vi "Unsubscribe.vi"(7 "Close if last?":bool, 8 "error in (no error)":errorcluster, 10 "Receivers Enqueuer":refnum<class "Message Enqueuer.lvclass">, 11 "Pub Sub Message Channel in":refnum<class "Pub Sub Message Channel.lvclass">) -> (0 "error out":errorcluster, 3 "Pub Sub Message Channel out":refnum<class "Pub Sub Message Channel.lvclass">)   [LabVIEW 2020, in "Actor Pub Sub Channels.lvlib" / "Pub Sub Message Channel.lvclass"]
uses:
  Pub Sub Message Channel.lvclass
  <vilib>/ActorFramework/Message Enqueuer/Message Enqueuer.lvclass
  Pub Sub Message Channel.lvclass/Pub Sub Message Channel.ctl
  <vilib>/ActorFramework/Message Queue/Message Queue.lvclass/Message Queue.ctl
  PubSub Status Reciever Interface Messages/Recieve Unsubscription Msg/Recieve Unsubscription Msg.lvclass/Recieve Unsubscription Msg.ctl
  <vilib>/ActorFramework/Message Enqueuer/Message Enqueuer.lvclass/Message Enqueuer.ctl
  <vilib>/ActorFramework/Message Enqueuer/Enqueue.vi
  PubSub Status Reciever Interface Messages/Recieve Unsubscription Msg/Recieve Unsubscription Msg.lvclass
  C:/Program Files/National Instruments/LabVIEW 2020/vi.lib/ActorFramework/Message/Message.lvclass
  <vilib>/ActorFramework/Message Priority Queue/Priority Enqueue.vi
  <vilib>/ActorFramework/Message Queue/Message Queue.lvclass
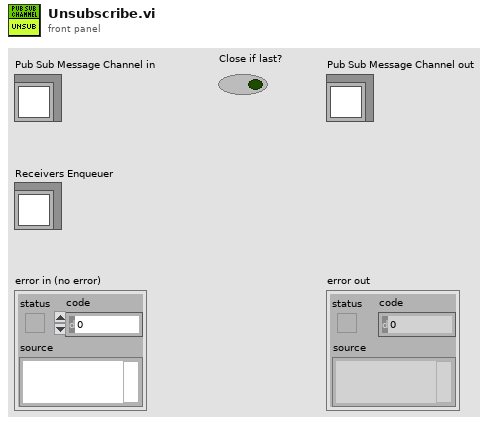
[diagram p1: front panel]
types:
  T1 = map{refnum<class "Message Enqueuer.lvclass">, string}
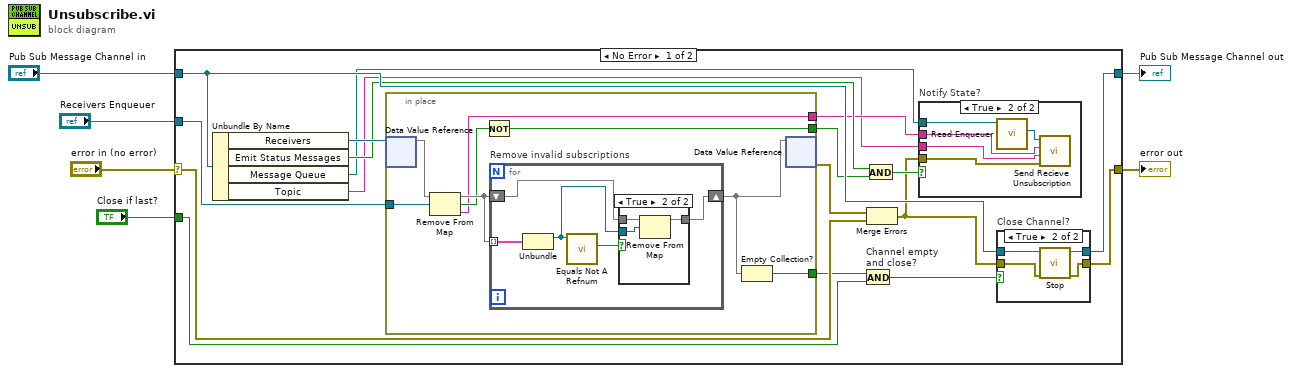
[diagram p0: block diagram]
diagram:
  n1 = case shown="No Error" "error in (no error)" {
    selector: "error in (no error)" -> [w23 w53]
    tunnel: [w19 w53] -> w5
    tunnel: [w18 w52] -> w3
    tunnel: "Pub Sub Message Channel in" -> [w17 w52]
    tunnel: "Receivers Enqueuer" -> [w21 _]
    tunnel: "Close if last?" -> [w14 _]
    frame No Error {
      n2 = Unbundle By Name(w17) -> ("Receivers"=w22:refnum<data-value>, "Emit Status Messages"=w11:bool, "Message Queue"=w10:refnum<class "Message Queue.lvclass">, "Topic"=w8:string)
      n3 = in-place {
        in-place-border: w21 -> [w40]
        in-place-border: [w42] -> w16
        in-place-border: [w35] -> w13
        in-place-border: [w36] -> w9
        n4 = in-place-dvr #1(w22) -> (w41:T1)  [unwired: 1 out]
        n5 = Remove From Map(10:w40, 11:w41) -> (1:w36:string, 2:w37:bool, 3:w38:T1)
        n6 = Not(x=w37) -> (.not. x?=w35:bool)
        n7 = for "Remove invalid subscriptions" {
          tunnel: w38 -> [w47] mode=indexing
          shift-right: [w45] -> w39
          shift-left: w38 -> [w46]
          n8 = Unbundle(w47) -> ("Message Enqueuer"=w44:refnum<class "Message Enqueuer.lvclass">)  [unwired: 1 out]
          n9 = call <vilib>:"Equals Not A Refnum.vi"("Message Enqueuer"=w44) -> ("Not a refnum?"=w43:bool)  [unwired: 10 in]
          n10 = case shown="True" w43 {
            tunnel: w46 -> [w48 w51]
            tunnel: [w48 w50] -> w45
            tunnel: w44 -> [_ w49]
            frame False {
            }
            frame True {
              n11 = Remove From Map(10:w49, 11:w51) -> (3:w50:T1)  [unwired: 2 out]
            }
          }
        }
        n12 = Empty Collection?(1:w39) -> (0:w42:bool)
        n13 = in-place-dvr #1(w39) -> (w20:errorcluster)  [unwired: 1 out]
      }
      n14 = And "Channel empty\nand close?"(x=w16, y=w14) -> (x .and. y?=w15:bool)
      n15 = And(x=w11, y=w13) -> (x .and. y?=w12:bool)
      n16 = Merge Errors(w20, w23) -> (w7:errorcluster)
      n17 = case "Notify State?" shown="True" w12 {
        tunnel: w10 -> [_ w28]
        tunnel: w9 -> [_ w26]
        tunnel: w8 -> [_ w25]
        tunnel: w7 -> [_ w24]
        frame False {
        }
        frame True {
          n18 = call <vilib>:"Read Enqueuer.vi"("Message Queue"=w28) -> ("Message Enqueuer"=w27:refnum<class "Message Enqueuer.lvclass">)  [unwired: 10 in]
          n19 = call "Send Recieve Unsubscription.vi"("error in (no error)"=w24, "Topic"=w25, "Name"=w26, "Message Enqueuer"=w27) -> ()  [unwired: 6 in, 2 out]
        }
      }
      n20 = case "Close Channel?" shown="True" w15 {
        tunnel: w7 -> [w29 w34]
        tunnel: [w29 w33] -> w19
        tunnel: [w30 w32] -> w18
        tunnel: w17 -> [w30 w31]
        frame False {
        }
        frame True {
          n21 = call "Stop.vi"("error in (no error)"=w34, "Pub Sub Message Channel in"=w31) -> ("error out"=w33:errorcluster, "Pub Sub Message Channel out"=w32:refnum<class "Pub Sub Message Channel.lvclass">)  [unwired: 8 in]
        }
      }
    }
    frame Error {
    }
  }
  "error out" <- w5
  "Pub Sub Message Channel out" <- w3
